vi "SLM_InvSinc.vi"(1 "LUT":dbl[](array[numeric]), 2 "Argument":dbl) -> (0 "InvSinc":dbl)   [LabVIEW 2024]
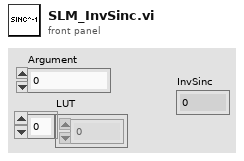
[diagram p1: front panel]
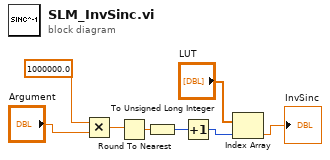
[diagram p0: block diagram]
diagram:
  n1 = Multiply(x=1000000.0, y="Argument") -> (x*y=w6:dbl)
  n2 = Round To Nearest(number=w6) -> (nearest integer value=w5:dbl)
  n3 = To Unsigned Long Integer(number=w5) -> (unsigned 32bit integer=w4:u32)
  n4 = Increment(x=w4) -> (x+1=w3:u32)
  n5 = Index Array(array="LUT", index=w3) -> (element=→"InvSinc":dbl)
